vi "EnFlo_Inlet_Heaters.vi"() -> ()   [LabVIEW 2010]
uses:
  ADAM Controls/Update_scan_value.ctl
panel:
  out "Zone Number":i32[](array[numeric])
  in  "Global Change":bool
  out "Messages":string
  in  "OK":bool
  in  "Zone On?":bool[](array[boolean])
  out "Current Temp":dbl[](array[numeric]) format="%.2f"
  in  "Set Point":dbl[](array[numeric]) format="%.2f"
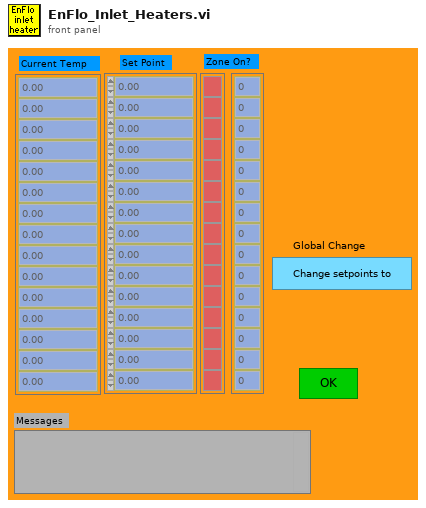
[diagram p1: front panel]
types:
  T1 = typedef "Update_scan_value.ctl" = cluster{"Channel Name":string, "New Value":dbl}
  T2 = typedef "Ch_description_ADAM.ctl" = cluster{"Ch Name":string, "Type":T3, "Function":T4, "Ch State":T5, "Calibration type":T6, "A":dbl, "B":dbl, "C":dbl, "D":dbl, "Comments":string, "Address":T7, "String":string, "Duty":u16}
  T3 = typedef "Module_type_ADAM.ctl" = enum16{"4011", "4012", "4013", "4014", "4016", "4017", "4018", "4021", "4050", "4052", "4053", "4060", "4080", "5000", "5017", "5018", "5024", "5051", "5056", "5060", "6060", "Tracker", "WEST", "GILL", "JEM", "VICI", "Vaisala", "DRUCK", "Run VI Named:", "IR2100", "PPT", "Comparator", "VIRTUAL", "Hold Value", "Read A", "Read Ch", "Coded", "Client Info", "Web Client", "X10", "Test"}
  T4 = typedef "Function_ADAM.ctl" = enum16{"Analogue Input", "Digital Input", "Event counter", "Event rate", "Analogue Output", "Digital Output", "Relay Output"}
  T5 = typedef "Channel_State.ctl" = enum16{"On", "Off", "Always On", "Always Off"}
  T6 = typedef "Calib_type_ADAM.ctl" = enum16{"Raw", "Bx + A", "Cx^2 + Bx + A", "Dx^3 + Cx^2 + Bx + A", "In Band", "Hi-Tec Q", "Hi-Tec M_dot", "Text"}
  T7 = typedef "Address.ctl" = cluster{"Main":i32, "Ch.":i32, "Sub":i32, "Port Name":string}
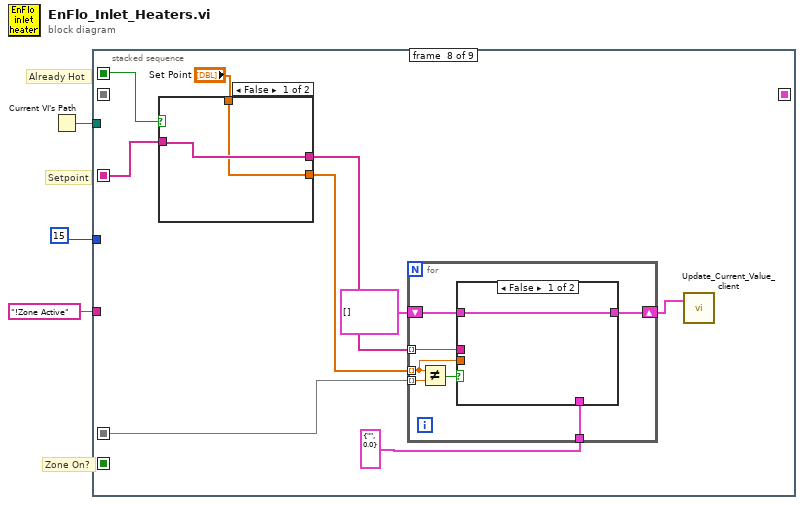
[diagram p0: block diagram]
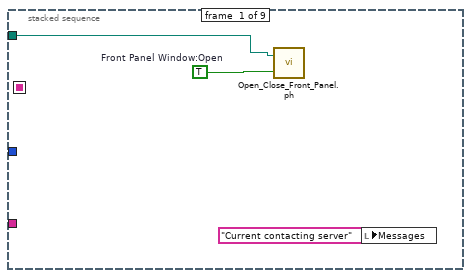
[diagram p2: hidden frame]
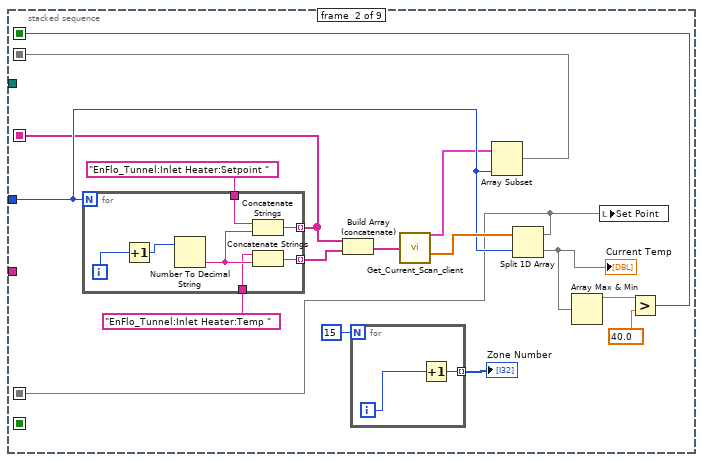
[diagram p3: hidden frame]
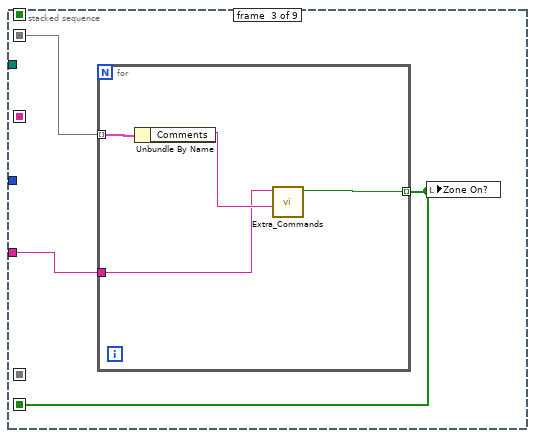
[diagram p4: hidden frame]
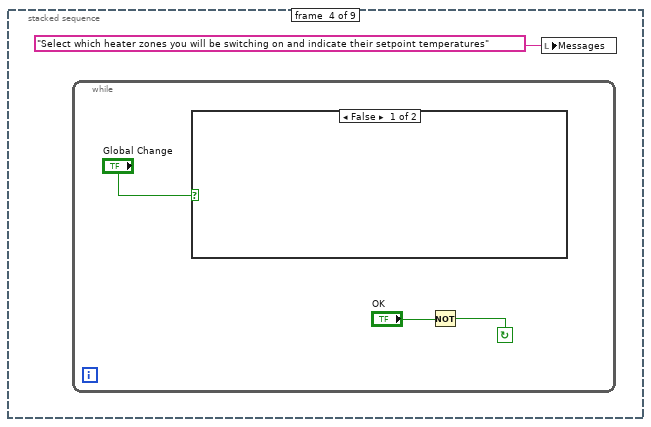
[diagram p5: hidden frame]
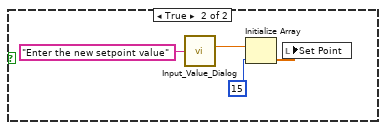
[diagram p6: hidden frame]
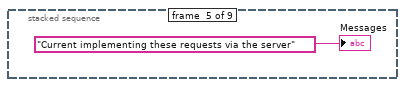
[diagram p7: hidden frame]
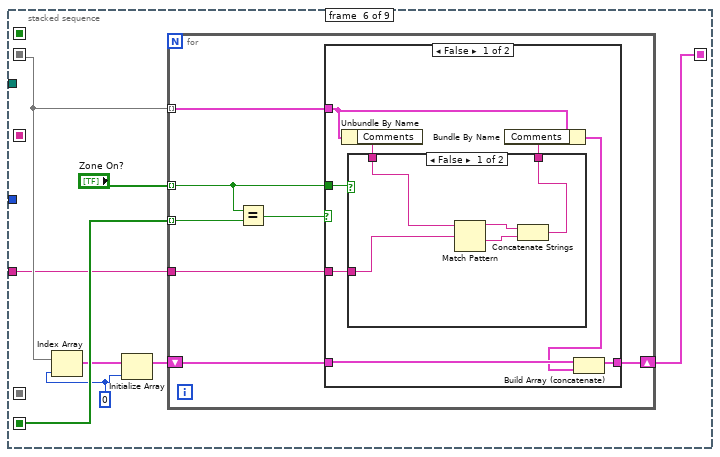
[diagram p8: hidden frame]
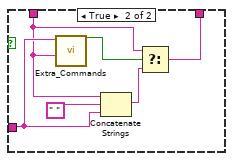
[diagram p9: hidden frame]
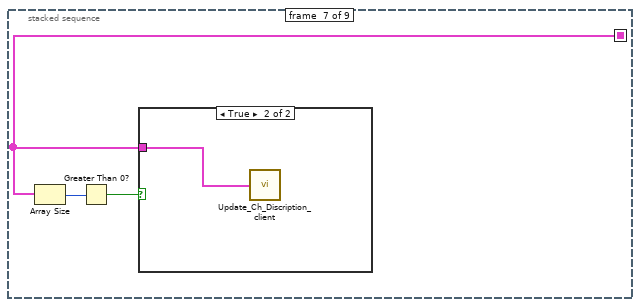
[diagram p11: hidden frame]
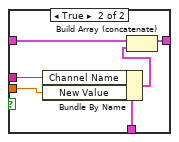
[diagram p13: hidden frame]
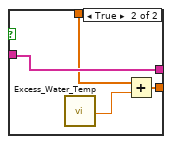
[diagram p14: hidden frame]
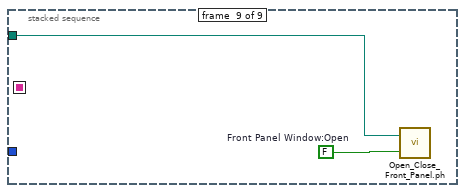
[diagram p15: hidden frame]
diagram:
  # "Already Hot"
  # "Zone On?"
  # "Setpoint"
  n1 = Current VI's Path() -> (path=w1:path)
  n2 = stacked-sequence {
    seq-local: [_ w15 _ _ _ _ _ _ _] -> [_ _ w34 _ _ w50 _ _ _]
    seq-local: [_ w14 _ _ _ _ _ _ _] -> [_ _ _ _ _ _ _ w95 _]
    seq-local: [_ _ w32 _ _ _ _ _ _] -> [_ _ _ _ _ w55 _ _ _]
    seq-local: [_ _ _ _ _ w51 _ _ _] -> [_ _ _ _ _ _ w83 _ _]
    seq-local: [_ w10 _ _ _ _ _ _ _] -> [_ _ _ _ _ _ _ w94 _]
    seq-local: [_ w7 _ _ _ _ _ _ _] -> [_ _ _ _ _ _ _ w92 _]
    tunnel: 15 -> [_ w17 _ _ _ _ _ _ _]
    tunnel: "!Zone Active" ("Command") -> [_ _ w33 _ _ w49 _ _ _]
    tunnel: w1 -> [w5 _ _ _ _ _ _ _ w116]
    frame #0 {
      w4 = TRUE  # Front Panel Window:Open
      n3 = call "Open_Close_Front_Panel.ph.vi"("Front Panel Window:Open"=w4, "VI path"=w5) -> ()  [unwired: 2 out]
      n4 = local write "Messages"("Current contacting server" ("Messages")) -> ()
    }
    frame #1 {
      n5 = for {
        N: w17 -> [_]
        tunnel: "EnFlo_Tunnel:Inlet Heater:Temp " -> [w28]
        tunnel: "EnFlo_Tunnel:Inlet Heater:Setpoint " -> [w27]
        tunnel: [w26] -> w14 mode=indexing
        tunnel: [w25] -> w20 mode=indexing
        i -> [w31]
        n6 = Increment(x=w31) -> (x+1=w30:i32)
        n7 = Number To Decimal String(number=w30) -> (decimal integer string=w29:string)  [unwired: 1 out]
        n8 = Concatenate Strings(w27, w29) -> (w26:string)
        n9 = Concatenate Strings(w28, w29) -> (w25:string)
      }
      n10 = Build Array (concatenate)(w14, w20) -> (w19:string[])
      n11 = for {
        N: 15 -> [_]
        tunnel: [w23] -> w8 mode=indexing
        i -> [w24]
        n12 = Increment(x=w24) -> (x+1=w23:i32)
      }
      "Zone Number" <- w8
      n13 = call "Get_Current_Scan_client.vi"("ADAM Ch Names"=w19) -> ("Ch Description Array"=w16:T2[], "Numerical Values"=w18:dbl[])  [unwired: 2 out]
      n14 = Array Subset(array=w16, length=w17) -> (w15:T2[])  [unwired: 1 in]
      n15 = Split 1D Array(array=w18, index=w17) -> (first subarray=w7:dbl[], second subarray=w13:dbl[])
      "Current Temp" <- w13
      n16 = Array Max & Min(array=w13) -> (max value=w12:dbl)  [unwired: 3 out]
      n17 = local write "Set Point"(w7) -> ()
      n18 = Greater?(x=w12, y=40.0) -> (0:w10:bool)
    }
    frame #2 {
      n19 = for {
        tunnel: w34 -> [w38] mode=indexing
        tunnel: w33 -> [w36]
        tunnel: [w35] -> w32 mode=indexing
        n20 = Unbundle By Name(w38) -> ("Comments"=w37:string)
        n21 = call "Extra_Commands.vi"("String to Search"=w37, "Command"=w36) -> ("Command Found"=w35:bool)  [unwired: 1 in, 4 out]
      }
      n22 = local write "Zone On?"(w32) -> ()
    }
    frame #3 {
      n23 = while {
        stop <- w41 continue-if-true
        n24 = case shown="False" "Global Change" {
          frame False {
          }
          frame True {
            n25 = call "Input_Value_Dialog.vi"("Message to user"="Enter the new setpoint value") -> ("Value received"=w44:dbl)  [unwired: 1 out]
            n26 = Initialize Array(w44, 15 ("Dimension Size")) -> (w43:dbl[])
            n27 = local write "Set Point"(w43) -> ()
          }
        }
        n28 = Not(x="OK") -> (.not. x?=w41:bool)
      }
      n29 = local write "Messages"("Select which heater zones you will be switching on and indicate their setpoint temperatures" ("Messages")) -> ()
    }
    frame #4 {
      "Messages" <- "Current implementing these requests via the server" ("Messages")
    }
    frame #5 {
      w54 = 0 ("Index")
      n30 = Index Array(array=w50, index=w54) -> (element=w53:T2)
      n31 = Initialize Array(w53, w54) -> (w52:T2[])
      n32 = for {
        shift-right: [w61] -> w51
        shift-left: w52 -> [w60]
        tunnel: "Zone On?" -> [w58] mode=indexing
        tunnel: w55 -> [w62] mode=indexing
        tunnel: w50 -> [w57] mode=indexing
        tunnel: w49 -> [w59]
        n33 = Equal?(x=w58, y=w62) -> (x = y?=w56:bool)
        n34 = case shown="False" w56 {
          tunnel: [w67 w82] -> w61
          tunnel: w60 -> [w69 w82]
          tunnel: w57 -> [w70 _]
          tunnel: w58 -> [w66 _]
          tunnel: w59 -> [w64 _]
          frame False {
            n35 = Unbundle By Name(w70) -> ("Comments"=w65:string)
            n36 = case shown="False" w66 {
              tunnel: w65 -> [w74 w78]
              tunnel: w64 -> [w75 w80]
              tunnel: [w71 w76] -> w63
              frame False {
                n37 = Match Pattern(string=w74, regular expression=w75) -> (before substring=w73:string, after substring=w72:string)  [unwired: 3 out]
                n38 = Concatenate Strings(w73, w72) -> (w71:string)
              }
              frame True {
                n39 = call "Extra_Commands.vi"("String to Search"=w78, "Command"=w80) -> ("Command Found"=w79:bool)  [unwired: 1 in, 4 out]
                n40 = Concatenate Strings(w78, " ", w80) -> (w77:string)
                n41 = Select(t=w78, s=w79, f=w77) -> (s? t:f=w76:string)
              }
            }
            n42 = Bundle By Name(cluster=w70, "Comments"=w63) -> (w68:T2)
            n43 = Build Array (concatenate)(w69, w68) -> (w67:T2[])
          }
          frame True {
          }
        }
      }
    }
    frame #6 {
      n44 = Array Size(array=w83) -> (size(s)=w85:i32)
      n45 = Greater Than 0?(x=w85) -> (x > 0?=w84:bool)
      n46 = case shown="True" w84 {
        tunnel: w83 -> [_ w86]
        frame False {
        }
        frame True {
          n47 = call "Update_Ch_Discription_client.vi"("Channels to update In"=w86) -> ()  [unwired: 1 out]
        }
      }
    }
    frame #7 {
      n48 = case shown="False" w94 {
        tunnel: w95 -> [w111 w115]
        tunnel: [w111 w115] -> w90
        tunnel: [w110 w112] -> w91
        tunnel: "Set Point" -> [w110 w113]
        frame False {
        }
        frame True {
          n49 = call "Excess_Water_Temp.vi"() -> ("Excess Temp"=w114:dbl)
          n50 = Add(x=w113, y=w114) -> (x+y=w112:dbl[])
        }
      }
      n51 = for {
        shift-right: [w97] -> w87
        shift-left: T1[] [] -> [w98]
        tunnel: w92 -> [w102] mode=indexing
        tunnel: w91 -> [w100] mode=indexing
        tunnel: w90 -> [w101] mode=indexing
        tunnel: T1 {"Channel Name"="", "New Value"=0.0} ("Update Scan Value Cluster") -> [w99]
        n52 = Not Equal?(x=w100, y=w102) -> (x != y?=w96:bool)
        n53 = case shown="False" w96 {
          tunnel: w101 -> [_ w109]
          tunnel: w100 -> [_ w108]
          tunnel: w99 -> [_ w106]
          tunnel: w98 -> [w103 w105]
          tunnel: [w103 w104] -> w97
          frame False {
          }
          frame True {
            n54 = Bundle By Name(cluster=w106, "Channel Name"=w109, "New Value"=w108) -> (w107:T1)
            n55 = Build Array (concatenate)(w105, w107) -> (w104:T1[])
          }
        }
      }
      n56 = call "Update_Current_Value_client.vi"("Update array in"=w87) -> ()  [unwired: 1 in]
    }
    frame #8 {
      w117 = FALSE  # Front Panel Window:Open
      n57 = call "Open_Close_Front_Panel.ph.vi"("Front Panel Window:Open"=w117, "VI path"=w116) -> ()  [unwired: 2 out]
    }
  }
